vi "VS SLSC Apply Static Properties.vi"(8 "error in (no error)":errorcluster, 9 "Configuration Data":T1, 10 "Refnum in":refnum<k21>, 11 "SLSC Module Name in":refnum<k21>) -> (0 "error out":errorcluster, 2 "Refnum out":refnum<k21>, 3 "SLSC Module Name out":refnum<k21>)   [LabVIEW 2015, in "SLSC-12201 DIO Engine.lvlib"]
uses:
  SLSC-12201 DIO Engine.lvlib
  <vilib>/SLSC/Set Generic Property (U64).vi
  <vilib>/SLSC/Set Generic Property (U32).vi
  <vilib>/SLSC/Set Generic Property (String).vi
  <vilib>/SLSC/Set Generic Property (I64).vi
  <vilib>/SLSC/Set Generic Property (I32).vi
  <vilib>/SLSC/Set Generic Property (DBL).vi
  <vilib>/SLSC/Set Generic Property (Bool).vi
  <vilib>/SLSC/Commit Properties for Devices.vi
  <vilib>/SLSC/SLSC.lvlib
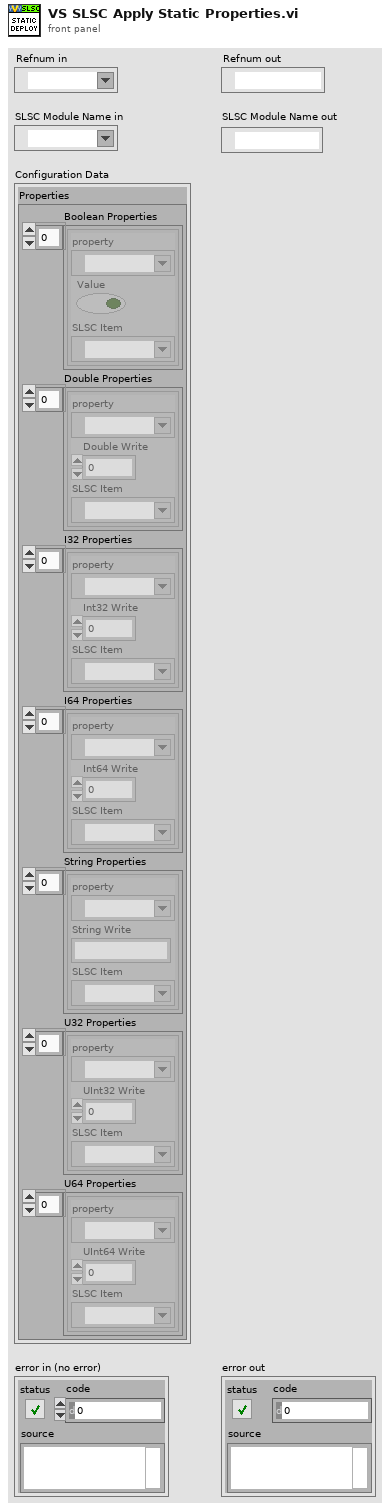
[diagram p1: front panel]
types:
  T1 = cluster{"Properties":cluster{"Boolean Properties":cluster{"property":refnum<k21>, "Value":bool, "SLSC Item":refnum<k21>}[], "Double Properties":cluster{"property":refnum<k21>, "Double Write":dbl, "SLSC Item":refnum<k21>}[], "I32 Properties":cluster{"property":refnum<k21>, "Int32 Write":i32, "SLSC Item":refnum<k21>}[], "I64 Properties":cluster{"property":refnum<k21>, "Int64 Write":i64, "SLSC Item":refnum<k21>}[], "String Properties":cluster{"property":refnum<k21>, "String Write":string, "SLSC Item":refnum<k21>}[], "U32 Properties":cluster{"property":refnum<k21>, "UInt32 Write":u32, "SLSC Item":refnum<k21>}[], "U64 Properties":cluster{"property":refnum<k21>, "UInt64 Write":u64, "SLSC Item":refnum<k21>}[]}}
  T2 = cluster{"property":refnum<k21>, "Value":bool, "SLSC Item":refnum<k21>}[]
  T3 = cluster{"property":refnum<k21>, "Double Write":dbl, "SLSC Item":refnum<k21>}[]
  T4 = cluster{"property":refnum<k21>, "Int32 Write":i32, "SLSC Item":refnum<k21>}[]
  T5 = cluster{"property":refnum<k21>, "Int64 Write":i64, "SLSC Item":refnum<k21>}[]
  T6 = cluster{"property":refnum<k21>, "String Write":string, "SLSC Item":refnum<k21>}[]
  T7 = cluster{"property":refnum<k21>, "UInt32 Write":u32, "SLSC Item":refnum<k21>}[]
  T8 = cluster{"property":refnum<k21>, "UInt64 Write":u64, "SLSC Item":refnum<k21>}[]
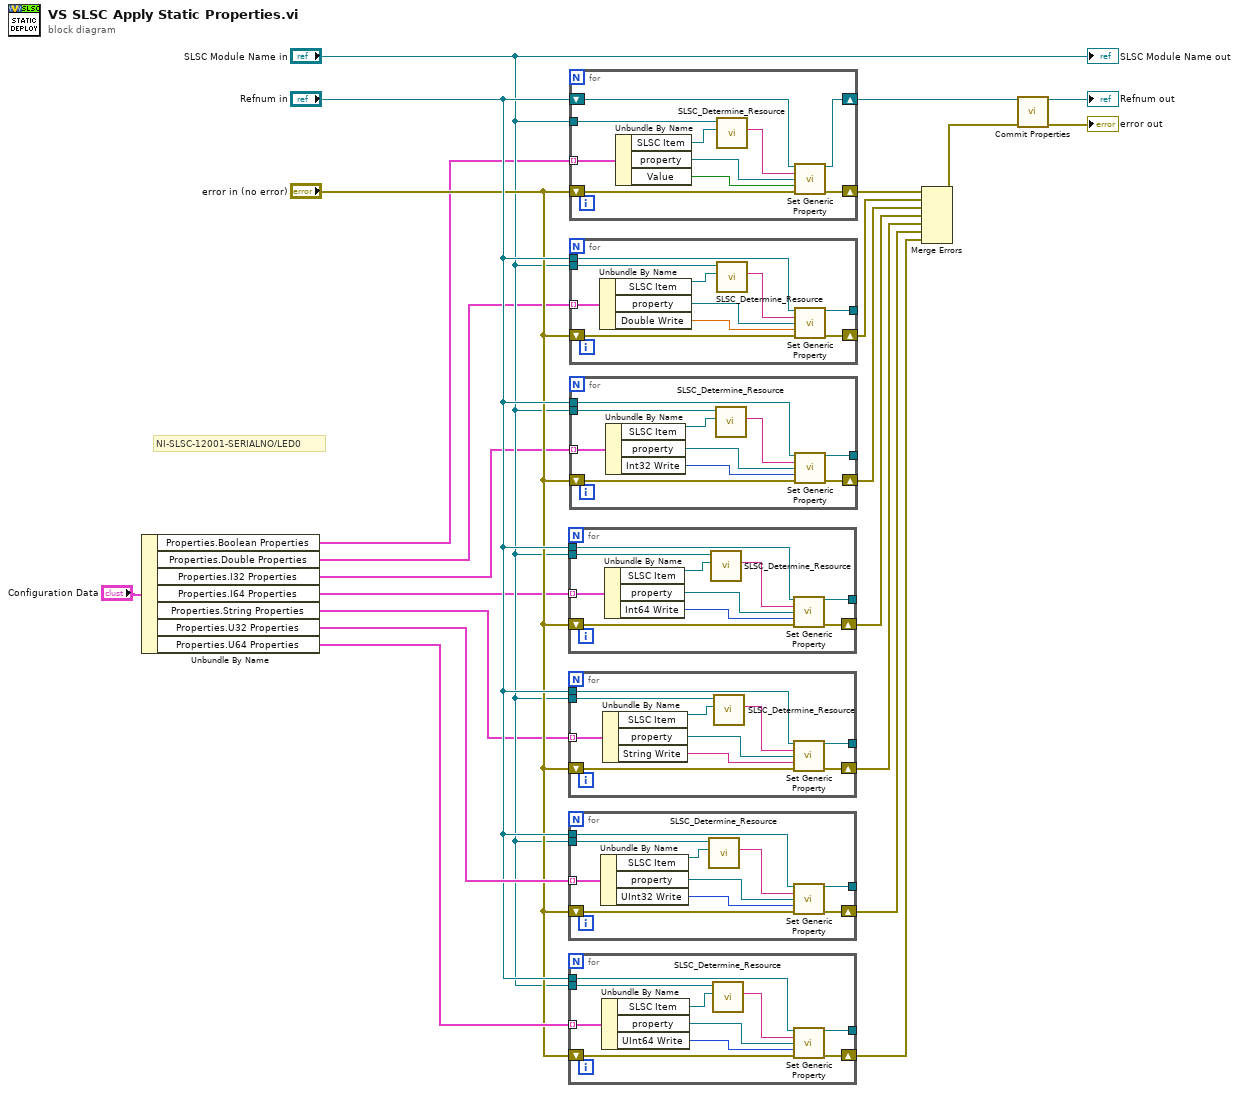
[diagram p0: block diagram]
diagram:
  # "NI-SLSC-12001-SERIALNO/LED0"
  n1 = Unbundle By Name("Configuration Data") -> ("Properties.Boolean Properties"=w5:T2, "Properties.Double Properties"=w7:T3, "Properties.I32 Properties"=w9:T4, "Properties.I64 Properties"=w10:T5, "Properties.String Properties"=w13:T6, "Properties.U32 Properties"=w18:T7, "Properties.U64 Properties"=w19:T8)
  n2 = for {
    tunnel: w10 -> [w32] mode=indexing
    tunnel: "Refnum in" -> [w26]
    tunnel: [w27] -> _
    shift-right: [w28] -> w12
    shift-left: "error in (no error)" -> [w29]
    tunnel: "SLSC Module Name in" -> [w24]
    n3 = Unbundle By Name(w32) -> ("SLSC Item"=w23:refnum<k21>, "property"=w31:refnum<k21>, "Int64 Write"=w30:i64)
    n4 = call "SLSC_Determine_Resource.vi"("SLSC Item"=w23, "SLSC Module Name"=w24) -> ("Resource"=w25:string)  [unwired: 9 in]
    n5 = call-poly <vilib>:"Set Generic Property.vi"("session in"=w26, "resources"=w25, "property"=w31, "property value"=w30, "error in (no error)"=w29) -> ("session out"=w27:refnum<k21>, "error out"=w28:errorcluster)  [unwired: 9 in]
  }
  n6 = for {
    tunnel: w13 -> [w42] mode=indexing
    tunnel: "Refnum in" -> [w36]
    tunnel: [w37] -> _
    shift-right: [w38] -> w14
    shift-left: "error in (no error)" -> [w39]
    tunnel: "SLSC Module Name in" -> [w35]
    n7 = Unbundle By Name(w42) -> ("SLSC Item"=w34:refnum<k21>, "property"=w41:refnum<k21>, "String Write"=w40:string)
    n8 = call "SLSC_Determine_Resource.vi"("SLSC Item"=w34, "SLSC Module Name"=w35) -> ("Resource"=w33:string)  [unwired: 9 in]
    n9 = call-poly <vilib>:"Set Generic Property.vi"("session in"=w36, "resources"=w33, "property"=w41, "property value"=w40, "error in (no error)"=w39) -> ("session out"=w37:refnum<k21>, "error out"=w38:errorcluster)  [unwired: 9 in]
  }
  n10 = for {
    tunnel: w18 -> [w52] mode=indexing
    tunnel: "Refnum in" -> [w46]
    tunnel: [w47] -> _
    shift-right: [w48] -> w20
    shift-left: "error in (no error)" -> [w49]
    tunnel: "SLSC Module Name in" -> [w45]
    n11 = Unbundle By Name(w52) -> ("SLSC Item"=w44:refnum<k21>, "property"=w51:refnum<k21>, "UInt32 Write"=w50:u32)
    n12 = call "SLSC_Determine_Resource.vi"("SLSC Item"=w44, "SLSC Module Name"=w45) -> ("Resource"=w43:string)  [unwired: 9 in]
    n13 = call-poly <vilib>:"Set Generic Property.vi"("session in"=w46, "resources"=w43, "property"=w51, "property value"=w50, "error in (no error)"=w49) -> ("session out"=w47:refnum<k21>, "error out"=w48:errorcluster)  [unwired: 9 in]
  }
  n14 = for {
    tunnel: w19 -> [w62] mode=indexing
    tunnel: "Refnum in" -> [w56]
    tunnel: [w57] -> _
    shift-right: [w58] -> w21
    shift-left: "error in (no error)" -> [w59]
    tunnel: "SLSC Module Name in" -> [w54]
    n15 = Unbundle By Name(w62) -> ("SLSC Item"=w55:refnum<k21>, "property"=w61:refnum<k21>, "UInt64 Write"=w60:u64)
    n16 = call "SLSC_Determine_Resource.vi"("SLSC Item"=w55, "SLSC Module Name"=w54) -> ("Resource"=w53:string)  [unwired: 9 in]
    n17 = call-poly <vilib>:"Set Generic Property.vi"("session in"=w56, "resources"=w53, "property"=w61, "property value"=w60, "error in (no error)"=w59) -> ("session out"=w57:refnum<k21>, "error out"=w58:errorcluster)  [unwired: 9 in]
  }
  n18 = for {
    tunnel: w5 -> [w72] mode=indexing
    shift-right: [w68] -> w6
    shift-left: "error in (no error)" -> [w69]
    tunnel: "SLSC Module Name in" -> [w65]
    shift-right: [w67] -> w2
    shift-left: "Refnum in" -> [w66]
    n19 = Unbundle By Name(w72) -> ("SLSC Item"=w64:refnum<k21>, "property"=w71:refnum<k21>, "Value"=w70:bool)
    n20 = call "SLSC_Determine_Resource.vi"("SLSC Item"=w64, "SLSC Module Name"=w65) -> ("Resource"=w63:string)  [unwired: 9 in]
    n21 = call-poly <vilib>:"Set Generic Property.vi"("session in"=w66, "resources"=w63, "property"=w71, "property value"=w70, "error in (no error)"=w69) -> ("session out"=w67:refnum<k21>, "error out"=w68:errorcluster)  [unwired: 9 in]
  }
  n22 = for {
    tunnel: w7 -> [w82] mode=indexing
    tunnel: "Refnum in" -> [w76]
    tunnel: [w77] -> _
    shift-right: [w78] -> w8
    shift-left: "error in (no error)" -> [w79]
    tunnel: "SLSC Module Name in" -> [w75]
    n23 = Unbundle By Name(w82) -> ("SLSC Item"=w73:refnum<k21>, "property"=w81:refnum<k21>, "Double Write"=w80:dbl)
    n24 = call "SLSC_Determine_Resource.vi"("SLSC Item"=w73, "SLSC Module Name"=w75) -> ("Resource"=w74:string)  [unwired: 9 in]
    n25 = call-poly <vilib>:"Set Generic Property.vi"("session in"=w76, "resources"=w74, "property"=w81, "property value"=w80, "error in (no error)"=w79) -> ("session out"=w77:refnum<k21>, "error out"=w78:errorcluster)  [unwired: 9 in]
  }
  n26 = for {
    tunnel: w9 -> [w92] mode=indexing
    tunnel: "Refnum in" -> [w86]
    tunnel: [w87] -> _
    shift-right: [w88] -> w11
    shift-left: "error in (no error)" -> [w89]
    tunnel: "SLSC Module Name in" -> [w85]
    n27 = Unbundle By Name(w92) -> ("SLSC Item"=w84:refnum<k21>, "property"=w91:refnum<k21>, "Int32 Write"=w90:i32)
    n28 = call "SLSC_Determine_Resource.vi"("SLSC Item"=w84, "SLSC Module Name"=w85) -> ("Resource"=w83:string)  [unwired: 9 in]
    n29 = call-poly <vilib>:"Set Generic Property.vi"("session in"=w86, "resources"=w83, "property"=w91, "property value"=w90, "error in (no error)"=w89) -> ("session out"=w87:refnum<k21>, "error out"=w88:errorcluster)  [unwired: 9 in]
  }
  n30 = Merge Errors(w6, w8, w11, w12, w14, w20, w21) -> (w3:errorcluster)
  n31 = call-poly <vilib>:"Commit Properties.vi"("session in"=w2, "error in (no error)"=w3) -> ("session out"=→"Refnum out":refnum<k21>, "error out"=→"error out":errorcluster)  [unwired: 12 in]
  "SLSC Module Name out" <- "SLSC Module Name in"
